vi "EMailErrors.vi"(11 "email":bool) -> (3 "Boolean":bool)   [LabVIEW 2012]
uses:
  <vilib>/Utility/sysdir.llb/System Directory Type.ctl
  <vilib>/Platform/browser.llb/Open URL in Default Browser (string).vi
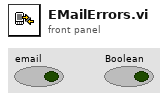
[diagram p1: front panel]
types:
  T1 = typedef "System Directory Type.ctl" = i32
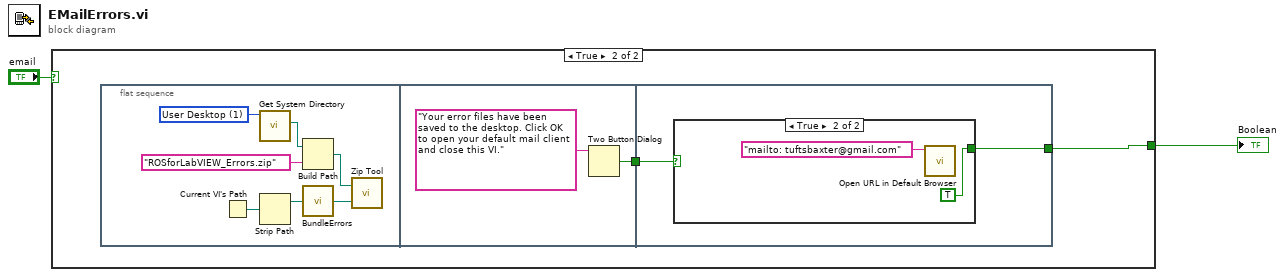
[diagram p0: block diagram]
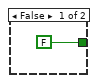
[diagram p2: hidden frame]
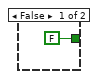
[diagram p3: hidden frame]
diagram:
  n1 = case shown="True" "email" {
    tunnel: [FALSE w4] -> w2
    frame False {
    }
    frame True {
      n2 = flat-sequence {
        tunnel: [w13] -> w5
        tunnel: w5 -> [w16]
        tunnel: [w15] -> w4
        frame #0 {
          w9 = T1 1 items=["User Home"=0, "User Desktop"=1, "User Documents"=2, "User Application Data"=3, "User Preferences"=4, "User Temporary"=5, "Public Documents"=6, "Public Application Data"=7, "Public Preferences"=8, "Public Cache"=13, "System Core Libraries"=9, "System Installed Libraries"=10, "Application Files"=11, "Boot Volume Root"=12] ("system directory type")
          n3 = Current VI's Path() -> (path=w11:path)
          n4 = call <vilib>:"Get System Directory.vi"("system directory type"=w9) -> ("system directory"=w7:path)  [unwired: 10 in]
          n5 = Strip Path(path=w11) -> (stripped path=w10:path)  [unwired: 1 out]
          n6 = Build Path(base path=w7, name or relative path="ROSforLabVIEW_Errors.zip") -> (appended path=w8:path)
          n7 = call <userlib>:"BundleErrors.vi"("base path"=w10) -> ("AllErrors"=w12:path)
          n8 = call "Zip Tool.vi"("Source File/Directory"=w12, "Target Zip File"=w8) -> ()  [unwired: 1 in]
        }
        frame #1 {
          n9 = Two Button Dialog(message="Your error files have been saved to the desktop. Click OK to open your default mail client and close this VI.") -> (T button?=w13:bool)  [unwired: 2 in]
        }
        frame #2 {
          n10 = case shown="True" w16 {
            tunnel: [FALSE TRUE] -> w15
            frame False {
            }
            frame True {
              n11 = call-poly <vilib>:"Open URL in Default Browser.vi"("URL"="mailto: tuftsbaxter@gmail.com") -> ()  [unwired: 5 in, 2 out]
            }
          }
        }
      }
    }
  }
  "Boolean" <- w2
